vi "SA Cond - Normalize wForms.vi"(0 "wForms IN":waveform(dbl)[](array[waveform]), 5 "Max of ALL Signals":dbl, 7 "Normalization Option":T1(ring)) -> (14 "wForms OUT":waveform(dbl)[](array[waveform]))   [LabVIEW 2020, in "GSwFormDSP.lvclass"]
uses:
  GSwFormDSP.lvclass
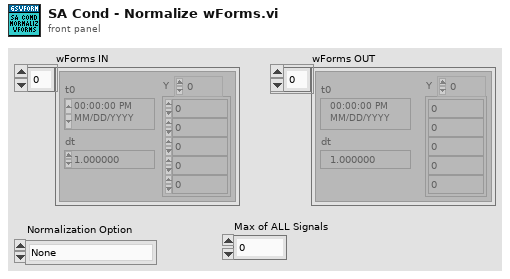
[diagram p1: front panel]
types:
  T1 = enum16{"None", "To itself", "To the max levels of ALL the signals"}
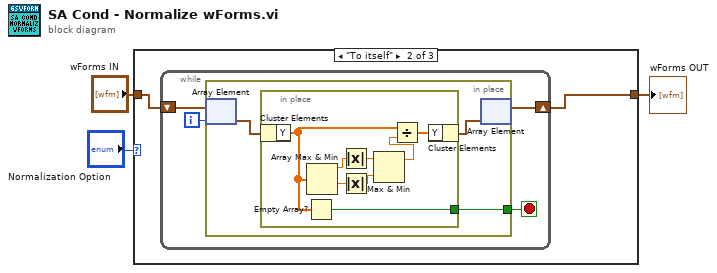
[diagram p0: block diagram]
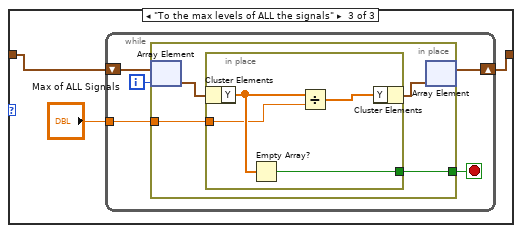
[diagram p3: hidden frame]
diagram:
  n1 = case shown="\"To itself\"" "Normalization Option" {
    tunnel: [w4 w5 w24] -> w2
    tunnel: "wForms IN" -> [w4 w6 w23]
    frame "None", Default {
    }
    frame "To itself" {
      n2 = while {
        shift-right: [w8] -> w5
        shift-left: w6 -> [w10]
        i -> [w9]
        stop <- w7 stop-if-true
        n3 = in-place {
          in-place-border: [w11] -> w7
          n4 = in-place-array #1(w10, w9) -> (w13:waveform(dbl))
          n5 = in-place {
            in-place-border: [w21] -> w11
            n6 = in-place-cluster #2(w13) -> ("Y"=w16:dbl[])
            n7 = Empty Array?(array=w16) -> (empty?=w21:bool)
            n8 = Array Max & Min(array=w16) -> (max value=w19:dbl, min value=w20:dbl)  [unwired: 2 out]
            n9 = Absolute Value(x=w19) -> (abs(x)=w18:dbl)
            n10 = Absolute Value(x=w20) -> (abs(x)=w17:dbl)
            n11 = Max & Min(x=w18, y=w17) -> (max(x,y)=w15:dbl)  [unwired: 1 out]
            n12 = Divide(x=w16, y=w15) -> (x/y=w14:dbl[])
            n13 = in-place-cluster #2("Y"=w14) -> (w12:waveform(dbl))
          }
          n14 = in-place-array #1(w12) -> (w8:waveform(dbl)[])  [unwired: 1 out]
        }
      }
    }
    frame "To the max levels of ALL the signals" {
      n15 = while {
        shift-right: [w27] -> w24
        shift-left: w23 -> [w29]
        tunnel: "Max of ALL Signals" -> [w25]
        i -> [w28]
        stop <- w26 stop-if-true
        n16 = in-place {
          in-place-border: [w31] -> w26
          in-place-border: w25 -> [w30]
          n17 = in-place-array #3(w29, w28) -> (w33:waveform(dbl))
          n18 = in-place {
            in-place-border: [w36] -> w31
            in-place-border: w30 -> [w34]
            n19 = in-place-cluster #4(w33) -> ("Y"=w37:dbl[])
            n20 = Empty Array?(array=w37) -> (empty?=w36:bool)
            n21 = Divide(x=w37, y=w34) -> (x/y=w35:dbl[])
            n22 = in-place-cluster #4("Y"=w35) -> (w32:waveform(dbl))
          }
          n23 = in-place-array #3(w32) -> (w27:waveform(dbl)[])  [unwired: 1 out]
        }
      }
    }
  }
  "wForms OUT" <- w2
